vi "IdentifyEG_G_LockinVISA.vi"(8 "error in (no error)":errorcluster, 11 "VISA resource name":refnum<visa-resource-name>) -> (0 "error out":errorcluster, 1 "Identified":bool, 2 "Instrument Type":T1(ring), 3 "VISA resource name out":refnum<visa-resource-name>)   [LabVIEW 2015]
panel:
  out "data":string
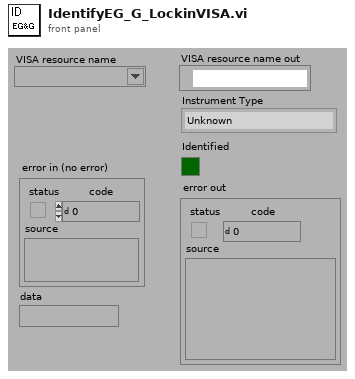
[diagram p1: front panel]
types:
  T1 = enum16{"Unknown", "SRS 850", "LR 700", "EG&G 5302", "EG&G 7260", "EG&G 7280", "AH 2500"}
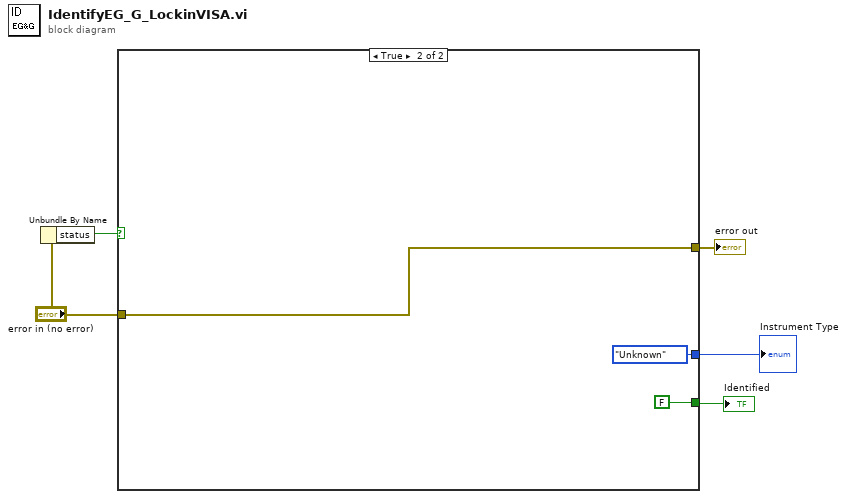
[diagram p0: block diagram]
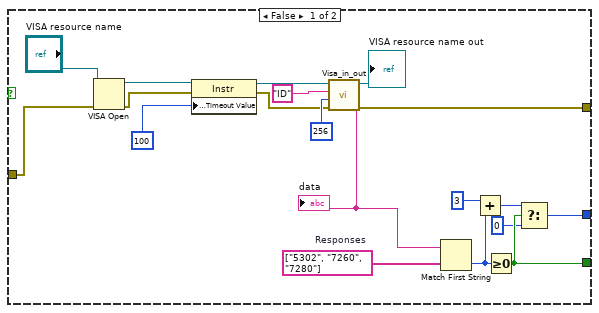
[diagram p2: hidden frame]
diagram:
  n1 = Unbundle By Name("error in (no error)") -> ("status"=w3:bool)
  n2 = case shown="True" w3 {
    tunnel: "error in (no error)" -> [w13 w27]
    tunnel: [w24 w27] -> w4
    tunnel: [w8 enum16{"Unknown", "EG&G 5302 Lockin"}."Unknown" ("Instrument")] -> w1
    tunnel: [w7 FALSE] -> w2
    frame False {
      w23 = string[] ["5302", "7260", "7280"]  # Responses
      n3 = VISA Open(error in (no error)=w13, VISA resource name="VISA resource name") -> (VISA resource name=w11:refnum<visa-resource-name>, error out=w10:errorcluster)  [unwired: 3 in]
      n4 = property class="Instr"(reference=w11, error in=w10, "General Settings:Timeout Value"=u32 100) -> (reference out=w17:refnum<visa-resource-name>, error out=w16:errorcluster)
      n5 = call "Visa_in_out.vi"("error in (no error)"=w16, "read count"=u32 256 ("byte count"), "write buffer"="ID", "VISA resource name"=w17) -> ("error out"=w24:errorcluster, "read buffer"=w20:string, "VISA resource name out"=→"VISA resource name out":refnum<visa-resource-name>)  [unwired: 5 in]
      "data" <- w20
      n6 = Match First String(2:w23, 3:w20) -> (0:w21:i32)  [unwired: 1 out]
      n7 = Add(x=3, y=w21) -> (x+y=w22:i32)
      n8 = Greater Or Equal To 0?(x=w21) -> (x >= 0?=w7:bool)
      n9 = Select(t=w22, s=w7, f=0) -> (s? t:f=w8:i32)
    }
    frame True {
    }
  }
  "error out" <- w4
  "Identified" <- w2
  "Instrument Type" <- w1
